vi "Create_Object.vi"(8 "error in (no error)":errorcluster, 9 "Terminal Map in":map{string, T1}(c390), 10 "owner refnum":variant, 11 "Boolean Constant in":refnum<class "Boolean Constant.lvclass">) -> (0 "error out":errorcluster, 1 "Terminal Map Out":map{string, T1}(c390), 3 "Boolean Constant out":refnum<class "Boolean Constant.lvclass">)   [LabVIEW 2025, in "Boolean Constant.lvclass"]
uses:
  Boolean Constant.lvclass
  C:/Users/mrjak/Documents/GitHub/LVGPT/LabVIEW/VIs/Classes/Node/Node.lvclass
  Terminal.ctl
  Node.lvclass/Node.ctl
  Constant.lvclass
  Node.lvclass
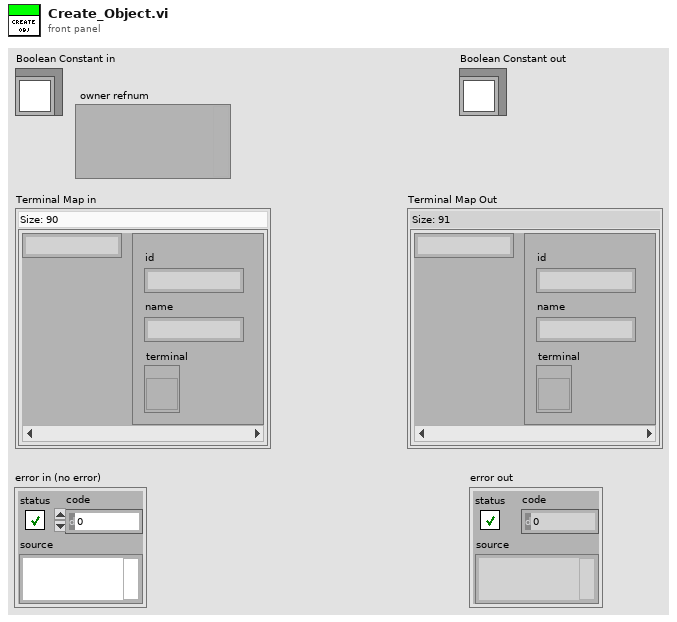
[diagram p1: front panel]
types:
  T1 = typedef "Terminal.ctl" = cluster{"id":string, "name":string, "terminal":refnum<vi>}
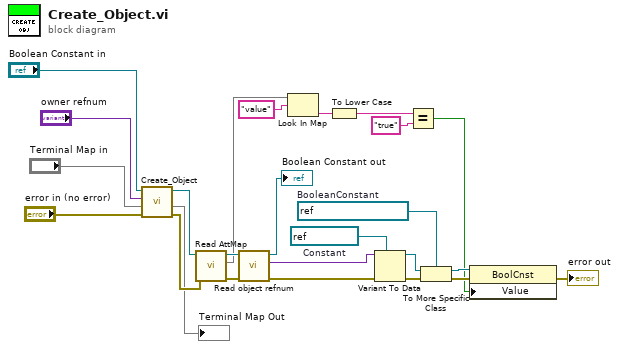
[diagram p0: block diagram]
diagram:
  w17 = refnum<vi> refnum  # BooleanConstant
  w18 = refnum<vi> refnum  # Constant
  n1 = call-parent "Create_Object.vi"("error in (no error)"="error in (no error)", "Terminal Map in"="Terminal Map in", "owner refnum"="owner refnum", "Constant in"="Boolean Constant in") -> ("error out"=w9:errorcluster, "Terminal Map Out"=→"Terminal Map Out":map{string, T1}, "Constant out"=w8:refnum<class "Boolean Constant.lvclass">)  [unwired: 5 in]
  n2 = call "Read AttMap.vi"("error in (no error)"=w9, "Node in"=w8) -> ("error out"=w21:errorcluster, "AttMap"=w4:map{string, string}, "Node out"=w20:refnum<class "Boolean Constant.lvclass">)  [unwired: 7 in]
  n3 = call-dynamic "Read object refnum.vi"("error in (no error)"=w21, "Node in"=w20) -> ("error out"=w7:errorcluster, "object refnum"=w3:variant, "Node out"=→"Boolean Constant out":refnum<class "Boolean Constant.lvclass">)  [unwired: 7 in]
  n4 = Look In Map(map=w4, key="value" ("valueConst")) -> (value=w12:string)  [unwired: 1 in, 1 out]
  n5 = To Lower Case(string=w12) -> (all lower case string=w1:string)
  n6 = Variant To Data(error in=w7, type=w18, Variant=w3) -> (data=w16:refnum<vi>, error out=w15:errorcluster)
  n7 = Equal?(x=w1, y="true" ("compareConst")) -> (x = y?=w10:bool)
  n8 = To More Specific Class(target class=w17, reference=w16, error in=w15) -> (specific class reference=w19:refnum<vi>, error out=w14:errorcluster)
  n9 = property class="BoolCnst"(reference=w19, error in=w14, "Value"=w10) -> (error out=→"error out":errorcluster)  [unwired: 1 out]
